vi "Initialize Tx Channel.vi"(7 "mode":u32(ring) items=["API429_TX_MODE_FRAMING", "API429_TX_MODE_LOOP", "API429_TX_MODE_PHYS_REPLAY", "API429_TX_MODE_FRAMING_DYNTAG", "API429_TX_MODE_FIFO", "API429_TX_MODE_RATE_CONTROLLED"], 8 "error in":errorcluster, 9 "channel speed":u32(ring) items=["API429_LO_SPEED", "API429_HI_SPEED"], 10 "channel number":u8, 11 "board handle":u8) -> (0 "error out":errorcluster, 2 "channel number out":u8, 3 "board handle out":u8)   [LabVIEW 2020, in "AIM ARINC 429 Hardware API.lvlib"]
uses:
  AIM ARINC 429 Hardware API.lvlib
  Channel Action.ctl
  <instrlib>/AIM GmbH/_ARINC-429/AIM429LV.lvlib
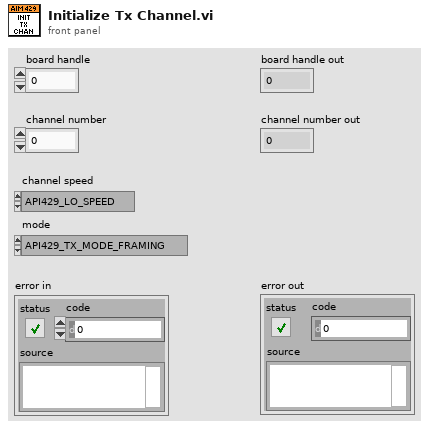
[diagram p1: front panel]
types:
  T1 = typedef "AIM ARINC 429 Hardware API.lvlib/Channel Action.ctl" = enum16{"Get Info", "Initialize", "Start", "Clear"}
  T2 = typedef "AIM ARINC 429 Hardware API.lvlib/Channel Status.ctl" = enum16{"Uninitialized", "Idle", "Active"}
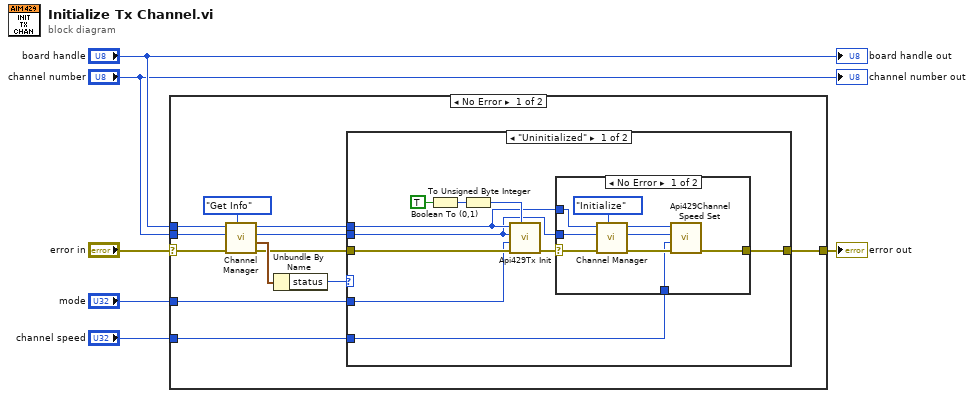
[diagram p0: block diagram]
diagram:
  n1 = case shown="No Error" "error in" {
    selector: "error in" -> [w10 w40]
    tunnel: "board handle" -> [w18 _]
    tunnel: "channel number" -> [w17 _]
    tunnel: [w9 w40] -> w3
    tunnel: "mode" -> [w8 _]
    tunnel: "channel speed" -> [w7 _]
    frame No Error {
      n2 = call "Channel Manager.vi"("action"=Channel_Action."Get Info", "error in"=w10, "channel number"=w17, "board handle"=w18) -> ("error out"=w13:errorcluster, "channel info"=w15:cluster{"count":u32, "status":T2}, "channel number out"=w11:u8, "board handle out"=w12:u8)  [unwired: 4 in]
      n3 = Unbundle By Name(w15) -> ("status"=w14:T2)
      n4 = case shown="\"Uninitialized\"" w14 {
        tunnel: w13 -> [w25 w39]
        tunnel: w12 -> [w22 _]
        tunnel: w11 -> [w21 _]
        tunnel: [w26 w39] -> w9
        tunnel: w8 -> [w20 _]
        tunnel: w7 -> [w19 _]
        frame "Uninitialized" {
          n5 = Boolean To (0,1)(Boolean=TRUE) -> (0, 1=w28:i16)
          n6 = To Unsigned Byte Integer(number=w28) -> (unsigned 8bit integer=w24:u8)
          n7 = call <instrlib>:"Api429Tx Init.vi"("auto_parity"=w24, "error in (no error)"=w25, "mode"=w20, "channel_id"=w21, "board_handle"=w22) -> ("error out"=w23:errorcluster)  [unwired: 6 in]
          n8 = case shown="No Error" w23 {
            selector: w23 -> [w36 w38]
            tunnel: [w32 w38] -> w26
            tunnel: w22 -> [w35 _]
            tunnel: w21 -> [w34 _]
            tunnel: w19 -> [w29 _]
            frame No Error {
              n9 = call "Channel Manager.vi"("action"=Channel_Action."Initialize", "error in"=w36, "channel number"=w34, "board handle"=w35) -> ("error out"=w33:errorcluster, "channel number out"=w30:u8, "board handle out"=w31:u8)  [unwired: 4 in, 1 out]
              n10 = call <instrlib>:"Api429Channel Speed Set.vi"("error in (no error)"=w33, "speed"=w29, "b_Chn"=w30, "board_handle"=w31) -> ("error out"=w32:errorcluster)  [unwired: 7 in]
            }
            frame Error {
            }
          }
        }
        frame Default {
          # "channel is already initialized; don't call init again"
        }
      }
    }
    frame Error {
    }
  }
  "error out" <- w3
  "board handle out" <- "board handle"
  "channel number out" <- "channel number"
